vi "WPI_IMU_ADIS16448_IMUAccumulation.vi"(1 "RESET?":bool, 2 "IMU Angle":dbl(knob) scale=-180.0..180.0) -> (0 "Accumulated Value":dbl)   [LabVIEW 2015, in "FRC_ADIS16448_IMU.lvlib"]
uses:
  FRC_ADIS16448_IMU.lvlib
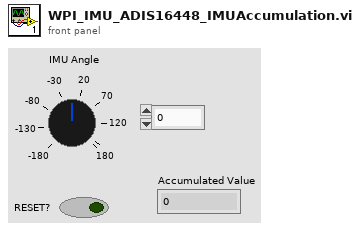
[diagram p1: front panel]
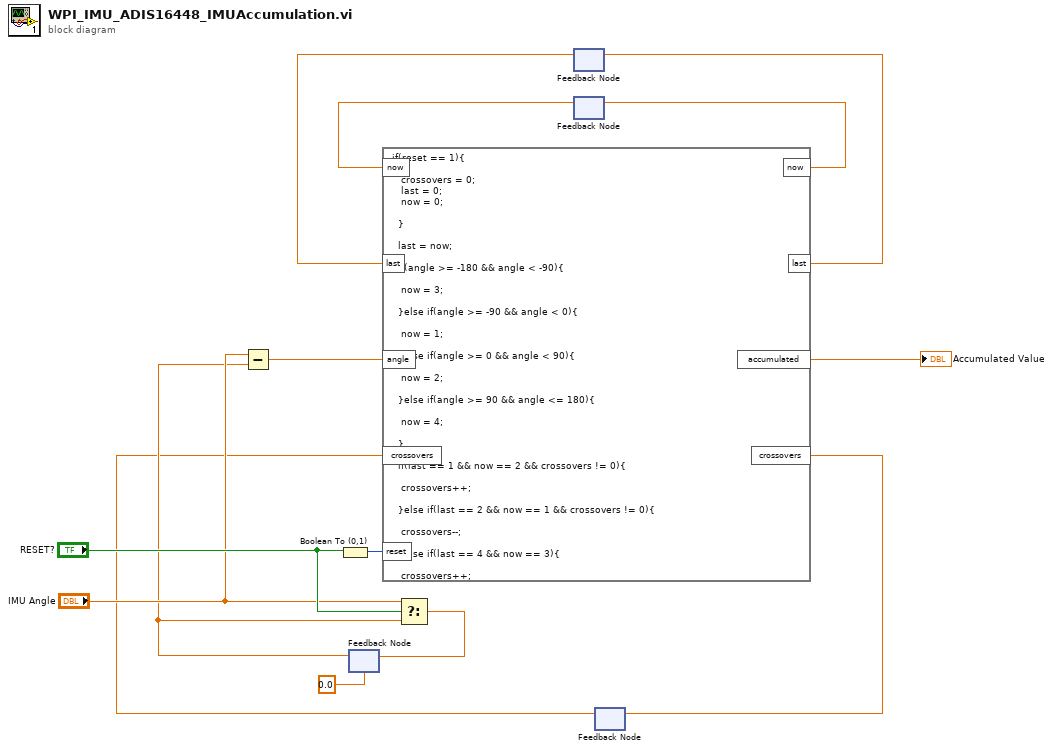
[diagram p0: block diagram]
diagram:
  n1 = Boolean To (0,1)(Boolean="RESET?") -> (0, 1=w13:i16)
  n2 = feedback #1(0.0 ("IMU Angle")) -> (w4:dbl)
  n3 = Subtract(x="IMU Angle", y=w4) -> (x-y=w10:dbl)
  n4 = Select(t="IMU Angle", s="RESET?", f=w4) -> (s? t:f=w5:dbl)
  n5 = feedback-in #1(w5) -> ()
  n6 = feedback #2() -> (w6:dbl)  [unwired: 1 in]
  n7 = feedback #3() -> (w8:dbl)  [unwired: 1 in]
  n8 = feedback #4() -> (w1:dbl)  [unwired: 1 in]
  n9 = formula code="if(reset == 1){\n\t\t\t\n\t\t\tcrossovers = 0;\n\t\t\tlast = 0;\n\t\t\tnow = 0;\n\t\t\t\n\t\t}\n\t\t\n\t\tlast = now;\n\t\t\n\t\tif(angle >= -180 && angle < -90){\n\t\t\t\n\t\t\tnow = 3;\n\t\t\t\n\t\t}else if(angle >= -90 && angle < 0){\n\t\t\t\n\t\t\tnow = 1;\n\t\t\t\n\t\t}else if(angle >= 0 && angle < 90){\n\t\t\t\n\t\t\tnow = 2;\n\t\t\t\n\t\t}else if(angle >= 90 && angle <= 180){\n\t\t\t\n\t\t\tnow = 4;\n\t\t\t\n\t\t}\n\t\t\n\t\tif(last == 1 && now == 2 && crossovers != 0){\n\t\t\t\n\t\t\tcrossovers++;\n\t\t\t\n\t\t}else if(last == 2 && now == 1 && crossovers != 0){\n\t\t\t\n\t\t\tcrossovers--;\n\t\t\t\n\t\t}else if(last == 4 && now == 3){\n\t\t\t\n\t\t\tcrossovers++;\n\t\t\t\n\t\t}else if(last == 3 && now == 4){\n\t\t\t\n\t\t\tcrossovers--;\n\t\t\t\n\t\t}\n\t\t\n\t\tint crossoverSign = (crossovers > 0) - (crossovers < 0); //Retrun 1 or -1 if it is not 0. If 0 it returns 0\n\t\tint angleSign = (angle > 0) - (angle < 0);\n\t\t\n  float accumulated = 0;\n\n\t\tif(crossoverSign == angleSign){\n\t\t\t\n\t\t\taccumulated = (180 * crossovers) + angle;\n\t\t\t\n\t\t}else if(crossoverSign == 1 && angleSign == -1){\n\t\t\t\n\t\t\taccumulated = (180 * crossovers) + abs(-180 - angle);\n\t\t\t\n\t\t}else if(crossoverSign == -1 && angleSign == 1){\n\t\t\t\n\t\t\taccumulated = (180 * crossovers) - abs(180 - angle);\n\t\t\t\n\t\t}else{ //If crossoverSign is 0 but angle sign is not there have been no crossovers but there is an angle change\n\t\t\t\n\t\t\taccumulated = angle;\n\t\t\t\n\t\t}"("angle"=w10, "reset"=w13, "last"=w6, "now"=w8, "crossovers"=w1) -> ("now"=w9:dbl, "last"=w7:dbl, "crossovers"=w2:dbl, "accumulated"=→"Accumulated Value":dbl)
  n10 = feedback-in #2(w7) -> ()
  n11 = feedback-in #3(w9) -> ()
  n12 = feedback-in #4(w2) -> ()
